vi "Clear Scan Time Out_2_test.vi"(6 "Channel number":i32, 7 "ESP32 ref":refnum<visa-resource-name>="COM4", 8 "error in (no error)":errorcluster, 11 "VISA Refnum in":refnum<visa-resource-name>) -> (0 "error out":errorcluster, 1 "error?":bool, 2 "Time out count":i32, 3 "VISA Refnum out":refnum<visa-resource-name>, 5 "ESP32 ref out":refnum<visa-resource-name>)   [LabVIEW 2023]
uses:
  <vilib>/Utility/error.llb/DialogType.ctl
panel:
  out "read buffer":string
  out "error out 3":errorcluster
  out "error out 2":errorcluster
  out "Measurements 3":dbl[](array[numeric])
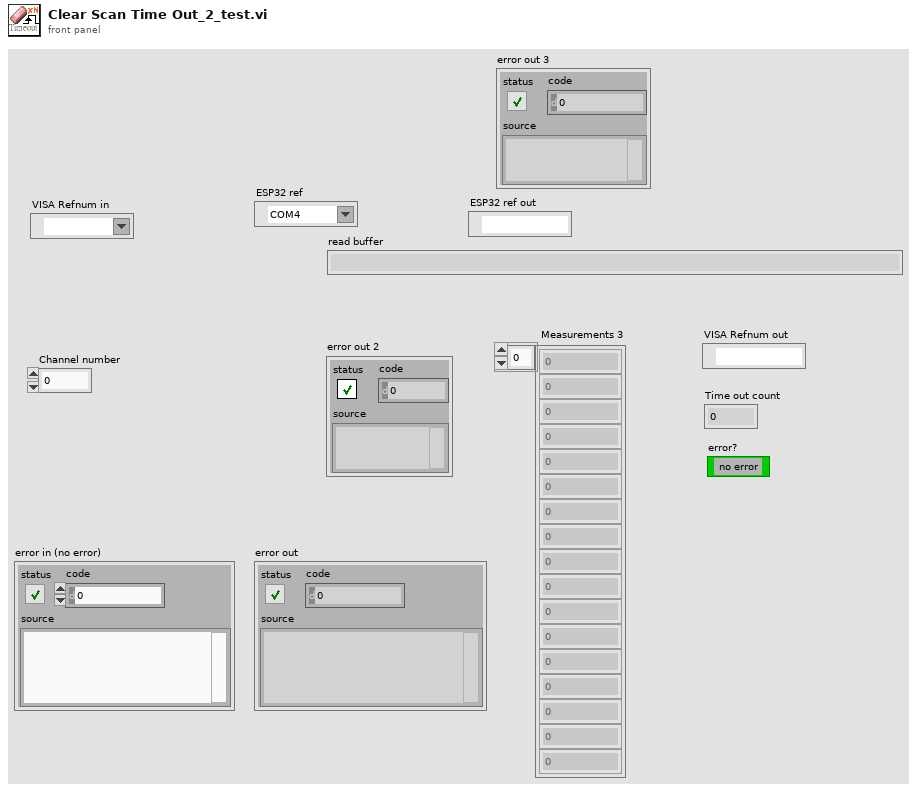
[diagram p1: front panel]
types:
  T1 = typedef "DialogType.ctl" = u16
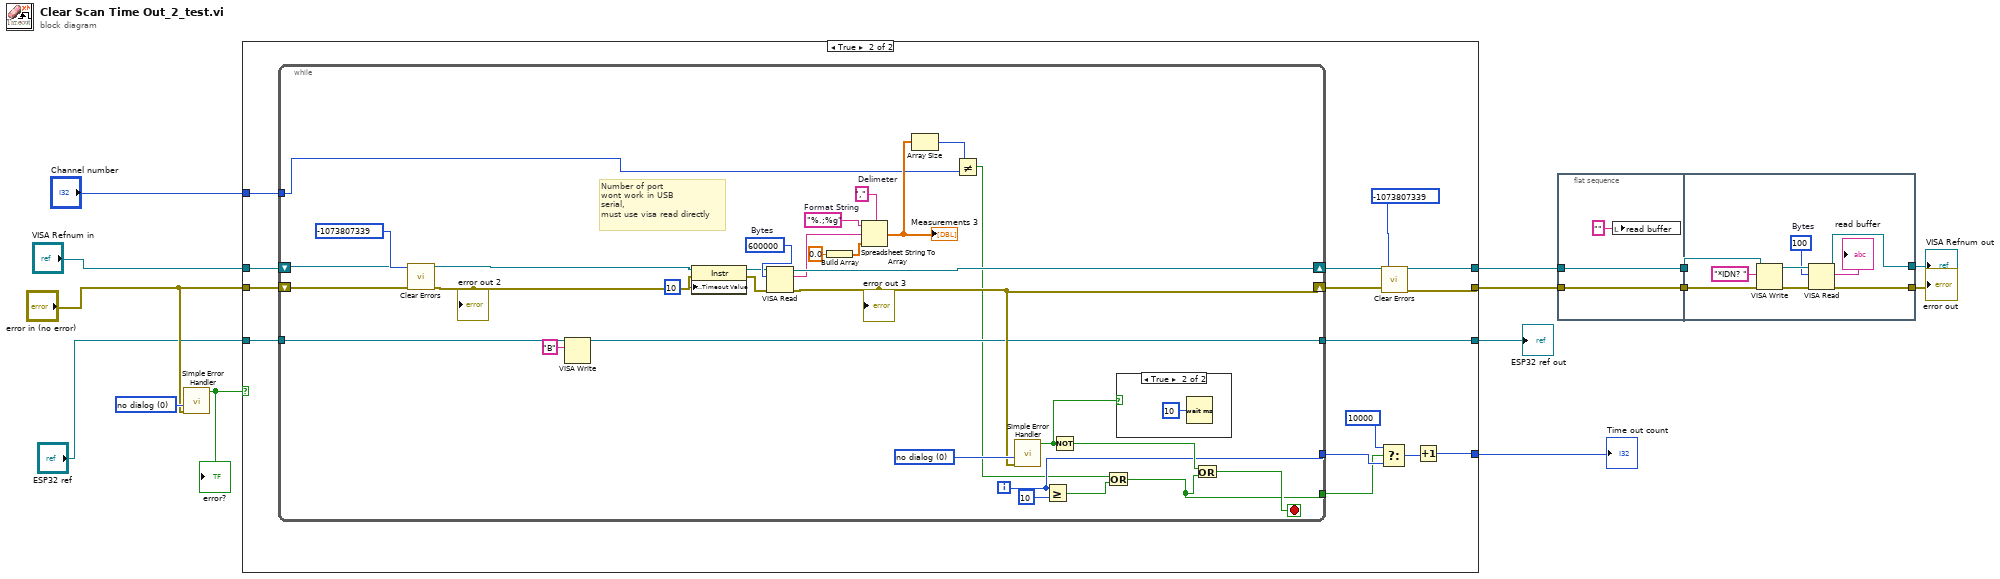
[diagram p0: block diagram]
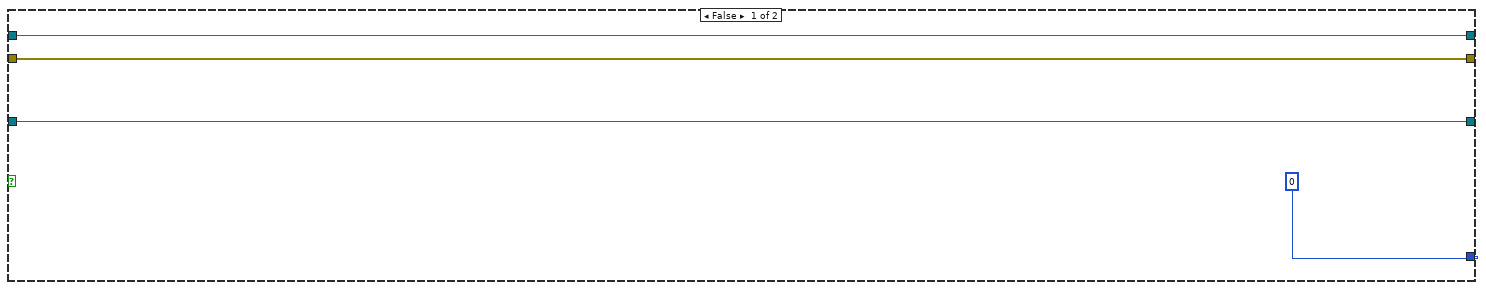
[diagram p2: hidden frame]
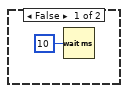
[diagram p3: hidden frame]
diagram:
  w13 = T1 0 items=["no dialog", "OK message", "continue or stop message", "OK message + warnings", "continue/stop + warnings"] ("type of dialog (OK msg:1)")
  n1 = call <vilib>:"Simple Error Handler.vi"("type of dialog (OK msg:1)"=w13, "error in (no error)"="error in (no error)") -> ("error?"=w11:bool)  [unwired: 3 in, 4 out]
  "error?" <- w11
  n2 = case shown="True" w11 {
    tunnel: [w18 w32] -> w4
    tunnel: "error in (no error)" -> [w17 w31]
    tunnel: "VISA Refnum in" -> [w18 w30]
    tunnel: [w17 w20] -> w3
    tunnel: [0 w29] -> w10
    tunnel: "ESP32 ref" -> [w15 w24]
    tunnel: [w15 w23] -> w8
    tunnel: "Channel number" -> [_ w22]
    frame False {
    }
    frame True {
      n3 = while {
        shift-right: [w57] -> w21
        shift-left: w31 -> [w60]
        shift-right: [w62] -> w32
        shift-left: w30 -> [w41]
        tunnel: [w53] -> w27
        tunnel: [w34] -> w26
        tunnel: w24 -> [w40]
        tunnel: [w39] -> w23
        tunnel: w22 -> [w36]
        i -> [w53]
        stop <- w54 stop-if-true
        w49 = ","  # Delimeter
        w50 = "%.;%g"  # Format String
        w45 = u32 600000  # Bytes
        w58 = T1 0 items=["no dialog", "OK message", "continue or stop message", "OK message + warnings", "continue/stop + warnings"] ("type of dialog (OK msg:1)")
        # "Number of port\nwont work in USB \nserial,\nmust use visa read directly"
        n4 = call <vilib>:"Clear Errors.vi"("error in (no error)"=w60, "specific error code to clear (0: all)"=-1073807339 ("code out")) -> ("error out"=w59:errorcluster)  [unwired: 4 in, 1 out]
        "error out 2" <- w59
        n5 = VISA Write(VISA resource name=w40, write buffer="B") -> (VISA resource name out=w39:refnum<visa-resource-name>)  [unwired: 1 in, 2 out]
        n6 = property class="Instr"(reference=w41, error in=w59, "General Settings:Timeout Value"=u32 10) -> (reference out=w44:refnum<visa-resource-name>, error out=w43:errorcluster)
        n7 = VISA Read(VISA resource name=w44, byte count=w45, error in (no error)=w43) -> (VISA resource name out=w62:refnum<visa-resource-name>, read buffer=w46:string, error out=w57:errorcluster)  [unwired: 1 out]
        "error out 3" <- w57
        n8 = Build Array(0.0) -> (w47:dbl[])
        n9 = Spreadsheet String To Array(delimiter (Tab)=w49, format string=w50, spreadsheet string=w46, array type (2D Dbl)=w47) -> (array=w38:dbl[])
        "Measurements 3" <- w38
        n10 = Array Size(array=w38) -> (size(s)=w37:i32)
        n11 = Not Equal?(x=w37, y=w36) -> (x != y?=w33:bool)
        n12 = call <vilib>:"Simple Error Handler.vi"("type of dialog (OK msg:1)"=w58, "error in (no error)"=w57) -> ("error?"=w52:bool)  [unwired: 3 in, 4 out]
        n13 = Greater Or Equal?(x=w53, y=10) -> (x >= y?=w35:bool)
        n14 = Not(x=w52) -> (.not. x?=w55:bool)
        n15 = Or(x=w33, y=w35) -> (x .or. y?=w34:bool)
        n16 = case shown="True" w52 {
          frame False {
            n17 = Wait (ms)(milliseconds to wait=u32 10) -> ()  [unwired: 1 out]
          }
          frame True {
            n18 = Wait (ms)(milliseconds to wait=u32 10) -> ()  [unwired: 1 out]
          }
        }
        n19 = Or(x=w55, y=w34) -> (x .or. y?=w54:bool)
      }
      n20 = Select(t=10000, s=w26, f=w27) -> (s? t:f=w28:i32)
      n21 = call <vilib>:"Clear Errors.vi"("error in (no error)"=w21, "specific error code to clear (0: all)"=-1073807339 ("code out")) -> ("error out"=w20:errorcluster)  [unwired: 4 in, 1 out]
      n22 = Increment(x=w28) -> (x+1=w29:i32)
    }
  }
  "Time out count" <- w10
  "ESP32 ref out" <- w8
  n23 = flat-sequence {
    tunnel: w3 -> [w66]
    tunnel: w4 -> [w67]
    tunnel: [w67] -> w2
    tunnel: [w66] -> w1
    tunnel: [w71] -> w6
    tunnel: [w70] -> w5
    tunnel: w2 -> [w69]
    tunnel: w1 -> [w68]
    frame #0 {
      n24 = local write "read buffer"("" ("read buffer")) -> ()
    }
    frame #1 {
      w74 = u32 100  # Bytes
      n25 = VISA Write(VISA resource name=w69, write buffer="*IDN? ", error in (no error)=w68) -> (VISA resource name out=w75:refnum<visa-resource-name>, error out=w76:errorcluster)  [unwired: 1 out]
      n26 = VISA Read(VISA resource name=w75, byte count=w74, error in (no error)=w76) -> (VISA resource name out=w71:refnum<visa-resource-name>, read buffer=→"read buffer":string, error out=w70:errorcluster)  [unwired: 1 out]
    }
  }
  "error out" <- w5
  "VISA Refnum out" <- w6
